vi "子VI-查看某框-加入序号.vi"(0 "测量结果":dbl[][](array[numeric])) -> (9 "测量结果 3":dbl[][](array[numeric]))   [LabVIEW 2018]
panel:
  out "测量结果 2":dbl[][](array[numeric])
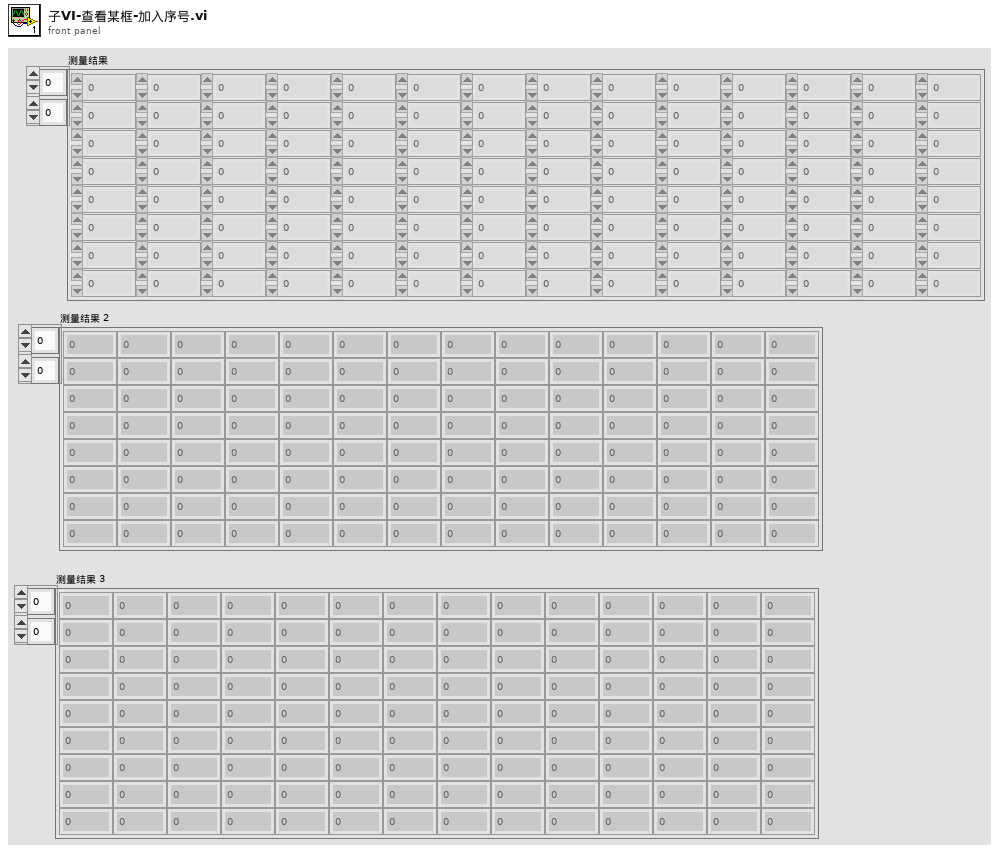
[diagram p1: front panel]
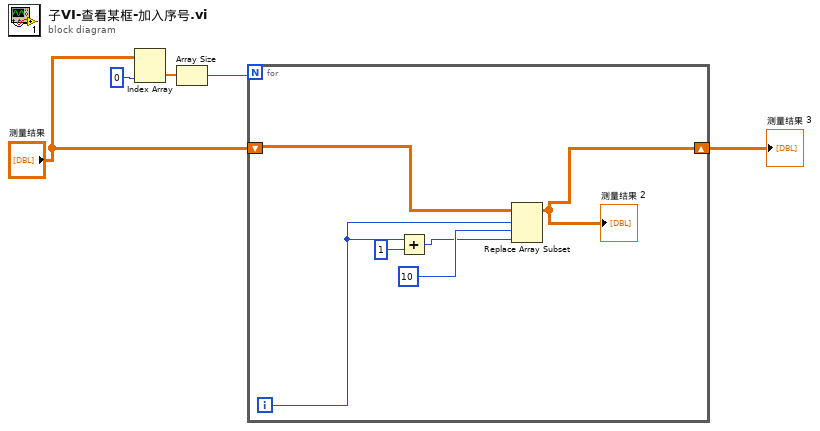
[diagram p0: block diagram]
diagram:
  n1 = Index Array(array="测量结果", index (col)=0 ("禁用的索引 (列)")) -> (element=w4:dbl[])  [unwired: 1 in]
  n2 = Array Size(array=w4) -> (size(s)=w2:i32)
  n3 = for {
    N: w2 -> [_]
    shift-right: [w9] -> w1
    shift-left: "测量结果" -> [w11]
    i -> [w8]
    n4 = Add(x=w8, y=1) -> (x+y=w7:i32)
    n5 = Replace Array Subset(array=w11, new element=w7, index (row)=w8, index (col)=10 ("禁用的索引 (列)")) -> (w9:dbl[][])
    "测量结果 2" <- w9
  }
  "测量结果 3" <- w1
